vi "VI Tree.vi"   [LabVIEW 2011, in "Tektronix 7000 Series.lvlib"]
doc: "This VI displays all the instrument driver VIs for the Tektronix TDS5k Series,TDS6k Series,TDS7k Series, DPO7k Series, DPO70k Series, DSA70k Series, MSO5k Series, DPO5k Series oscilloscopes. The block diagram window displays all the user-callable VIs of the instrument driver in an organized table."
uses:
  Tektronix 7000 Series.lvlib
  Data/Read (Single Waveform).vi
  Data/Read Waveform Measurement (Amplitude).vi
  Configure/Math/Configure Math Expression (Unary Operation).vi
  Configure/Configure Trigger (Edge).vi
  Data/Low Level/Fetch Waveform Measurement (More).vi
  Data/Low Level/Fetch (Waveform).vi
  Configure/Configure Bus Source (SPI-Data).vi
  Configure/Math/Configure Spectral (Magnitude).vi
  Configure/Math/Configure Math (Basic).vi
panel:
  # "Copyright 2006 - 2011 National Instruments Corporation.  ALL RIGHTS RESERVED."
  # "SEE DIAGRAM\nFOR VI TREE."
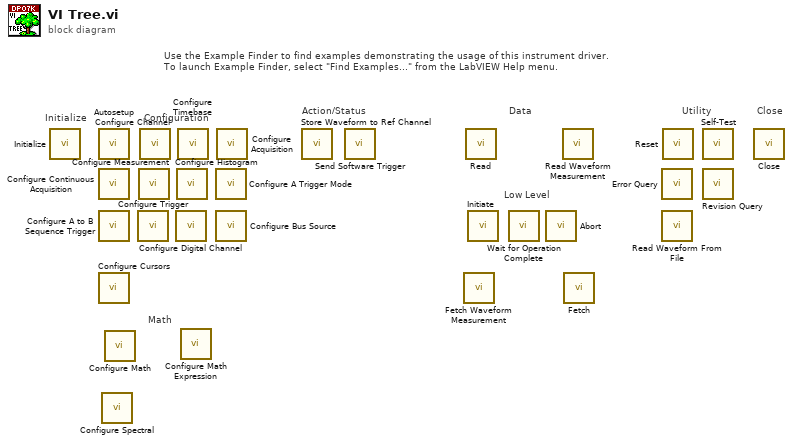
[diagram p0: block diagram]
diagram:
  # "Use the Example Finder to find examples demonstrating the usage of this instrument driver.\nTo launch Example Finder, select \"Find Examples...\" from the LabVIEW Help menu."
  # "Math"
  # "Low Level"
  # "Action/Status"
  # "Configuration"
  # "Utility"
  # "Data"
  # "Close"
  # "Initialize"
  n1 = call "Initialize.vi"() -> ()  [unwired: 10 in, 2 out]
  n2 = call "Autosetup.vi"() -> ()  [unwired: 10 in, 2 out]
  n3 = call "Configure Continuous Acquisition.vi"() -> ()  [unwired: 10 in, 2 out]
  n4 = call "Configure A to B Sequence Trigger.vi"() -> ()  [unwired: 14 in, 2 out]
  n5 = call "Configure Cursors.vi"() -> ()  [unwired: 14 in, 2 out]
  n6 = call-poly "Configure Spectral.vi"() -> ()  [unwired: 14 in, 2 out]
  n7 = call-poly "Configure Math.vi"() -> ()  [unwired: 10 in, 2 out]
  n8 = call-poly "Configure Trigger.vi"() -> ()  [unwired: 14 in, 2 out]
  n9 = call "Configure Measurement.vi"() -> ()  [unwired: 14 in, 2 out]
  n10 = call "Configure Channel.vi"() -> ()  [unwired: 14 in, 2 out]
  n11 = call "Configure Digital Channel.vi"() -> ()  [unwired: 10 in, 2 out]
  n12 = call "Configure Histogram.vi"() -> ()  [unwired: 14 in, 2 out]
  n13 = call "Configure Timebase.vi"() -> ()  [unwired: 10 in, 2 out]
  n14 = call-poly "Configure Math Expression.vi"() -> ()  [unwired: 9 in, 3 out]
  n15 = call "Configure A Trigger Mode.vi"() -> ()  [unwired: 14 in, 2 out]
  n16 = call-poly "Configure Bus Source.vi"() -> ()  [unwired: 10 in, 2 out]
  n17 = call "Configure Acquisition.vi"() -> ()  [unwired: 14 in, 2 out]
  n18 = call "Store Waveform to Ref Channel.vi"() -> ()  [unwired: 10 in, 2 out]
  n19 = call "Send Software Trigger.vi"() -> ()  [unwired: 10 in, 2 out]
  n20 = call-poly "Fetch Waveform Measurement.vi"() -> ()  [unwired: 13 in, 3 out]
  n21 = call-poly "Read.vi"() -> ()  [unwired: 9 in, 3 out]
  n22 = call "Initiate.vi"() -> ()  [unwired: 10 in, 2 out]
  n23 = call "Wait for Operation Complete.vi"() -> ()  [unwired: 10 in, 2 out]
  n24 = call "Abort.vi"() -> ()  [unwired: 10 in, 2 out]
  n25 = call-poly "Read Waveform Measurement.vi"() -> ()  [unwired: 13 in, 3 out]
  n26 = call-poly "Fetch.vi"() -> ()  [unwired: 9 in, 3 out]
  n27 = call "Error Query.vi"() -> ()  [unwired: 8 in, 4 out]
  n28 = call "Read Waveform From File.vi"() -> ()  [unwired: 10 in, 6 out]
  n29 = call "Reset.vi"() -> ()  [unwired: 10 in, 2 out]
  n30 = call "Self-Test.vi"() -> ()  [unwired: 8 in, 4 out]
  n31 = call "Revision Query.vi"() -> ()  [unwired: 8 in, 4 out]
  n32 = call "Close.vi"() -> ()  [unwired: 11 in, 1 out]
